vi "RTEH Classification to String.vi"(7 "Classification as Number":u32) -> (8 "Classification as String":string)   [LabVIEW 2017]
doc: "To avoid string manipulation the RTEH stores classifications as integers. This VI converts an integer into a 4 byte human readable string to make the classification easy to handle."
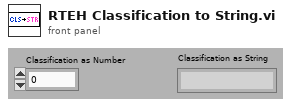
[diagram p1: front panel]
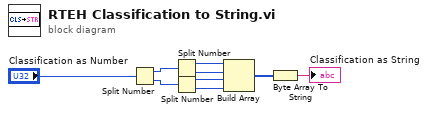
[diagram p0: block diagram]
diagram:
  n1 = Split Number(x="Classification as Number") -> (hi(x)=w8:u16, lo(x)=w7:u16)
  n2 = Split Number(x=w8) -> (hi(x)=w6:u8, lo(x)=w5:u8)
  n3 = Split Number(x=w7) -> (hi(x)=w4:u8, lo(x)=w3:u8)
  n4 = Build Array(w6, w5, w4, w3) -> (w2:u8[])
  n5 = Byte Array To String(unsigned byte array=w2) -> (string=→"Classification as String":string)
